vi "Do.vi"(8 "error in (no error)":errorcluster, 10 "Actor in":refnum<class "Actor.lvclass">, 11 "Broadcast DBL Msg In":refnum<class "Broadcast I32 Msg.lvclass">) -> (0 "error out":errorcluster, 2 "Actor out":refnum<class "Actor.lvclass">)   [LabVIEW 2015, in "Broadcast I32 Msg.lvclass"]
doc: "(<B>Filename</B>: Actor Framework.lvlib:Message.lvclass:Do.vi)\n\nDefines what a message does when it is received by an actor. Generally, a message instructs an actor to invoke one of its methods. By default, this method does nothing. A child class must override it to define behavior. Create a child class by using the Actor Framework Message Maker dialog box."
uses:
  Broadcast I32 Msg.lvclass
  <vilib>/ActorFramework/Actor/Actor.lvclass
  IViewable/IViewable.lvclass
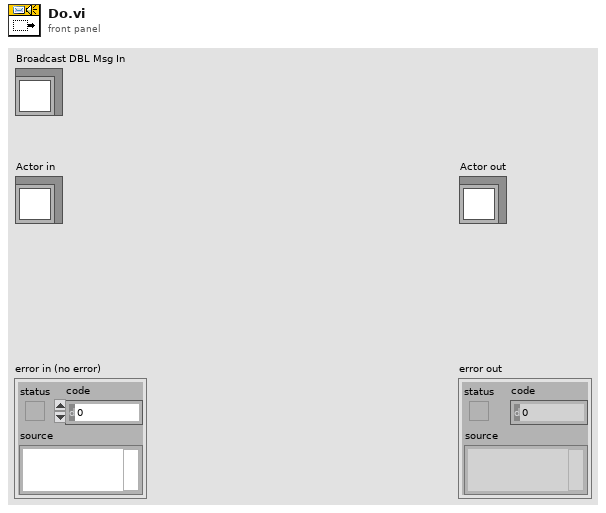
[diagram p1: front panel]
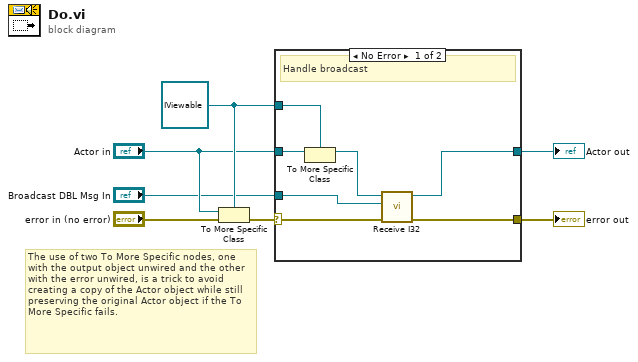
[diagram p0: block diagram]
diagram:
  w6 = refnum<class "IViewable.lvclass"> refnum ("Actor in")
  # "The use of two To More Specific nodes, one with the output object unwired and the other with the error unwired, is a trick to avoid creating a copy of the Actor object while still preserving the original Actor object if the To More Specific fails."
  n1 = To More Specific Class(target class=w6, reference="Actor in", error in="error in (no error)") -> (error out=w7:errorcluster)  [unwired: 1 out]
  n2 = case shown="No Error" w7 {
    selector: w7 -> [w12 w16]
    tunnel: [w11 w16] -> w5
    tunnel: [w10 w15] -> w4
    tunnel: "Actor in" -> [w14 w15]
    tunnel: w6 -> [w13 _]
    tunnel: "Broadcast DBL Msg In" -> [w9 _]
    frame No Error {
      # "Handle broadcast"
      n3 = To More Specific Class(target class=w13, reference=w14) -> (specific class reference=w8:refnum<class "IViewable.lvclass">)  [unwired: 1 in, 1 out]
      n4 = call-dynamic "Receive I32.vi"("error in (no error)"=w12, "Broadcast I32 Msg"=w9, "IViewable In"=w8) -> ("error out"=w11:errorcluster, "IViewable Out"=w10:refnum<class "IViewable.lvclass">)  [unwired: 7 in]
    }
    frame Error {
      # "If type check fails, pass the\noriginal object out again."
    }
  }
  "error out" <- w5
  "Actor out" <- w4
